vi "Analog Write.vi"   [LabVIEW 2014, in "LMH-LINX.lvlib"]
uses:
  <vilib>/MakerHub/LINX/LMH-LINX.lvlib
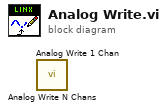
[diagram p0: block diagram]
diagram:
  n1 = call <vilib>:"Analog Write N Chans.vi"() -> ()  [unwired: 10 in, 2 out]
  n2 = call <vilib>:"Analog Write 1 Chan.vi"() -> ()  [unwired: 10 in, 2 out]
